vi "Quiz Scoreboard.vi"() -> ()   [LabVIEW 2025]
uses:
  Team.ctl
  State.ctl
  State Data.ctl
  <vilib>/DAQmx/create/channels.llb/DAQmx Create Channel (DI-Digital Input).vi
panel:
  out "Tab Control":enum32{"Setup", "Go"}(tab)
  in  "OK Button":bool
  in  "Team 1 Input":tag="Dev1/port0/line0" caption="Input"
  in  "Team 2 Input":tag="Dev1/port0/line1" caption="Input"
  in  "Team 3 Input":tag="Dev1/port0/line2" caption="Input"
  in  "Team 4 Input":tag="Dev1/port0/line3" caption="Input"
  in  "Team 1 Name":string="When I think about Yule I touch my Elf" caption="Team Name"
  in  "Team 2 Name":string="Bad Santa" caption="Team Name"
  in  "Team 3 Name":string="LabVIEWlots" caption="Team Name"
  in  "Team 4 Name":string="Operation Yule Tree" caption="Team Name"
  out "2D Picture":picture
  out "Team 4":T1
  out "Team 3":T1
  out "Team 2":T1
  out "Team 1":T1
  # "Team 1"
  # "Team 2"
  # "Team 3"
  # "Team 4"
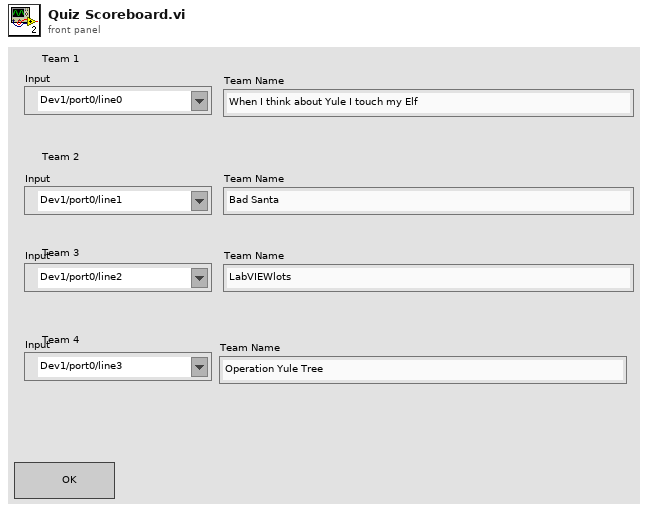
[diagram p1: front panel]
types:
  T1 = typedef "Team.ctl" = cluster{"ON":bool, "Name":bool, "Score":i32, "Split":string}
  T2 = typedef "State.ctl" = enum16{"Stop", "Initialize", "Wait for User Input", "Create DAQ Device"}
  T3 = typedef "State Data.ctl" = cluster{"Team 1":T1, "Team 2":T1, "Team 3":T1, "Team 4":T1, "Team Ref 1":refnum<vi>, "Team Ref 2":refnum<vi>, "Team Ref 3":refnum<vi>, "Team Ref 4":refnum<vi>, "Time":i32}
  T4 = typedef "eventvkey.ctl" = enum16{"ASCII", "Enter", "Return", "Shift", "Ctrl", "Alt", "Cmd", "Opt", "Caps", "NumLock", "Clear", "Break", "Up", "Down", "Left", "Right", "Insert", "Delete", "Home", "End", "PageUp", "PageDown", "Escape", "Help", "Pause", "ScrollLock", "F1", "F2", "F3", "F4", "F5", "F6", "F7", "F8", "F9", "F10", "F11", "F12", "F13", "F14", "F15", "F16", "F17", "F18", "F19", "F20", "F21", "F22", "F23", "F24", "Play", "VolumeUp", "VolumeDown", "Mute", "Two Byte Char"}
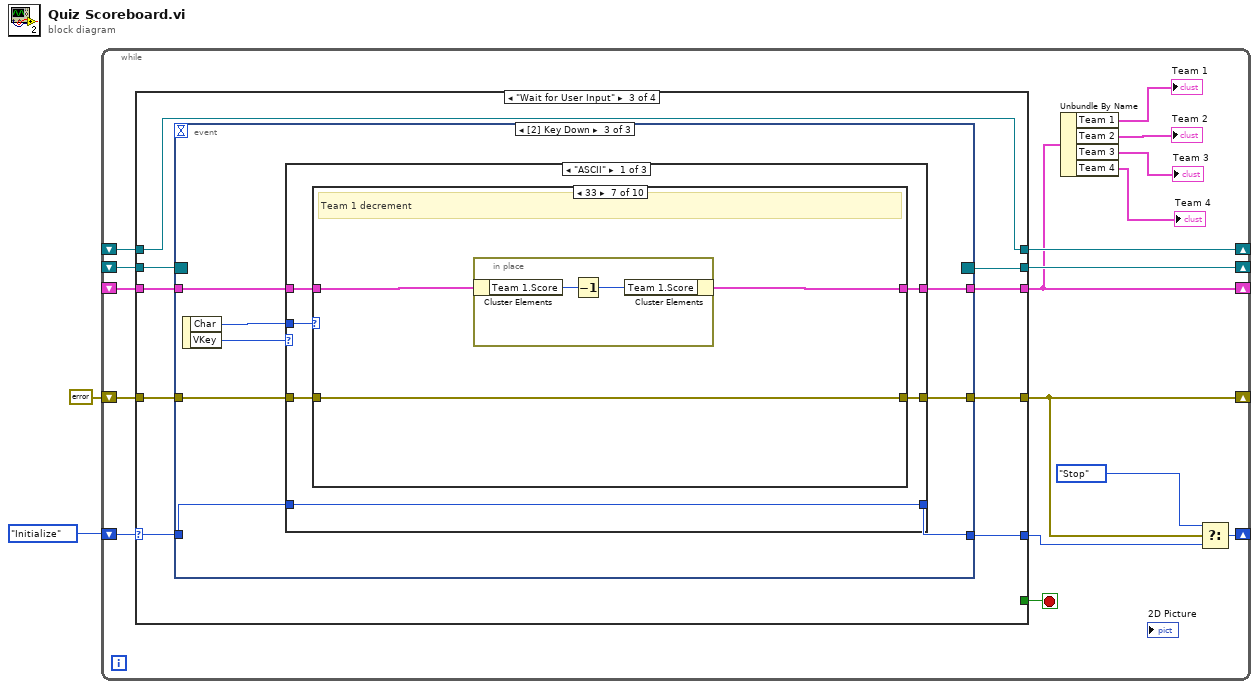
[diagram p0: block diagram]
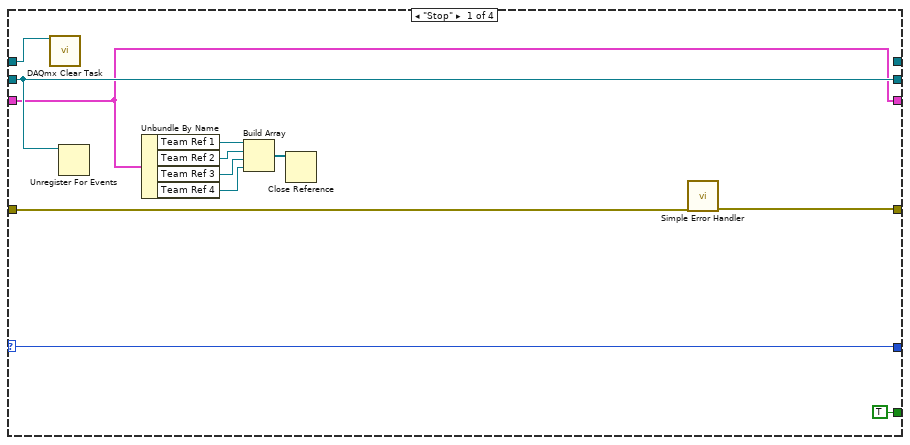
[diagram p2: hidden frame]
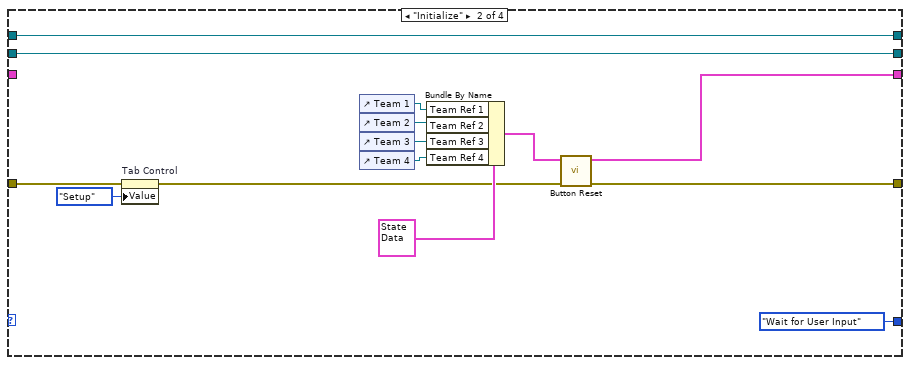
[diagram p3: hidden frame]
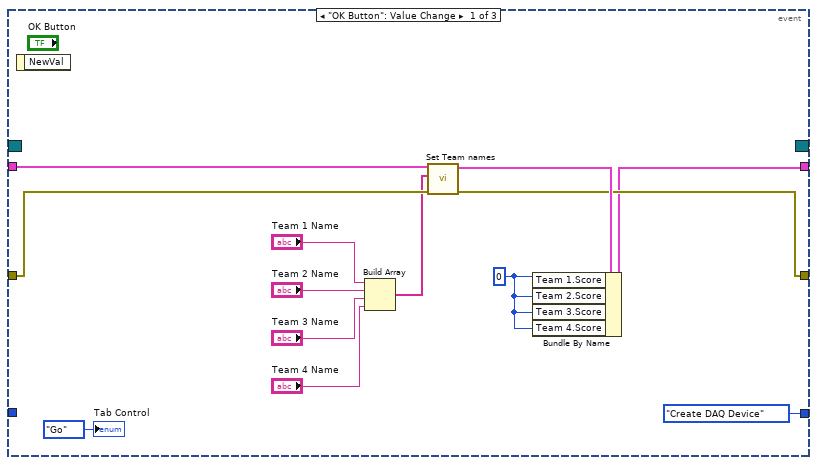
[diagram p4: hidden frame]
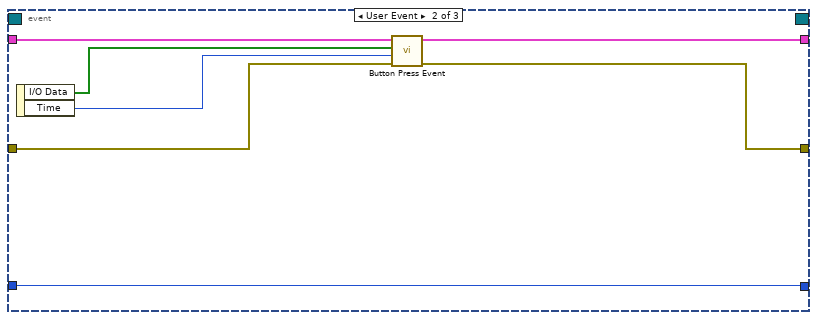
[diagram p5: hidden frame]
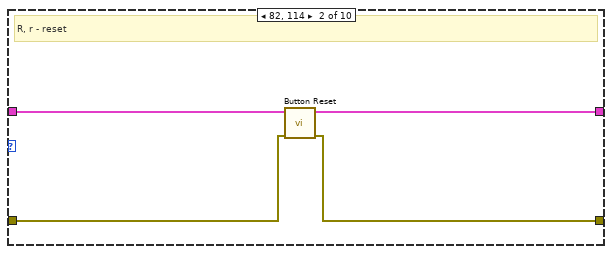
[diagram p7: hidden frame]
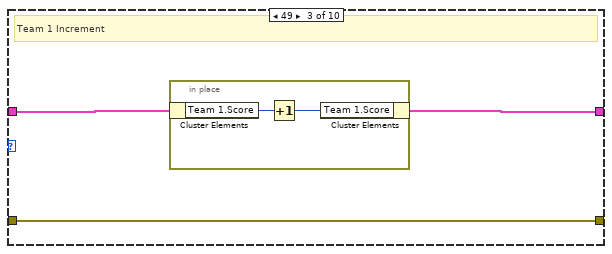
[diagram p8: hidden frame]
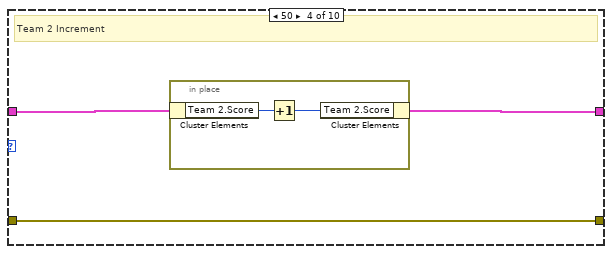
[diagram p9: hidden frame]
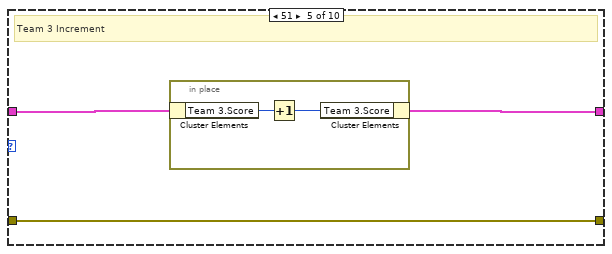
[diagram p10: hidden frame]
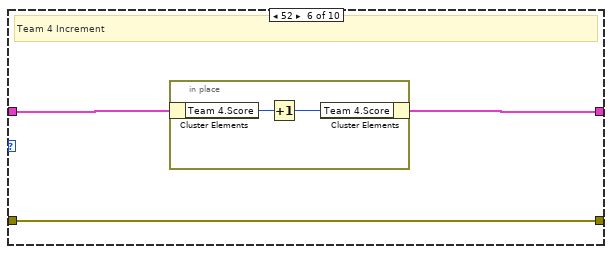
[diagram p11: hidden frame]
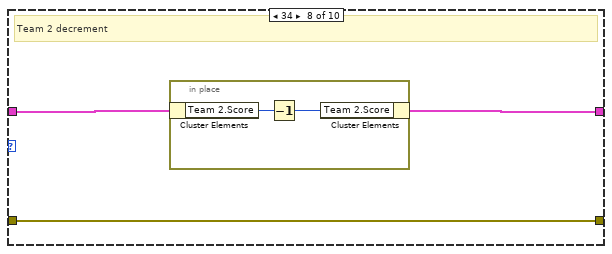
[diagram p12: hidden frame]
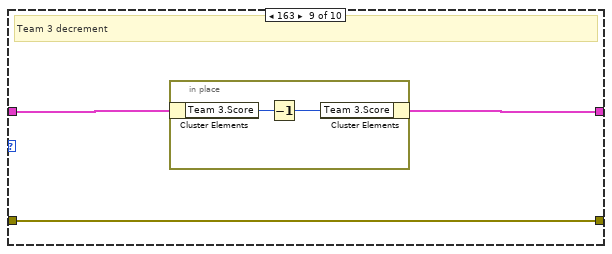
[diagram p13: hidden frame]
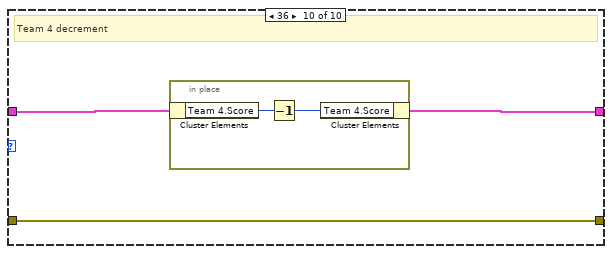
[diagram p14: hidden frame]
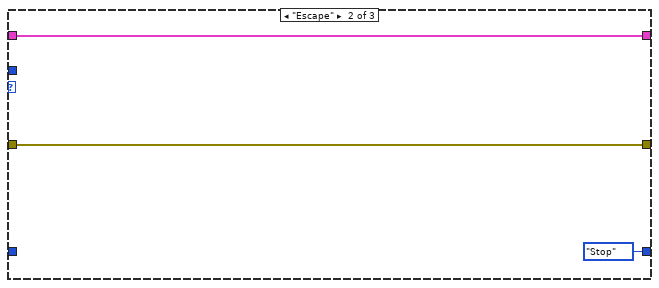
[diagram p15: hidden frame]
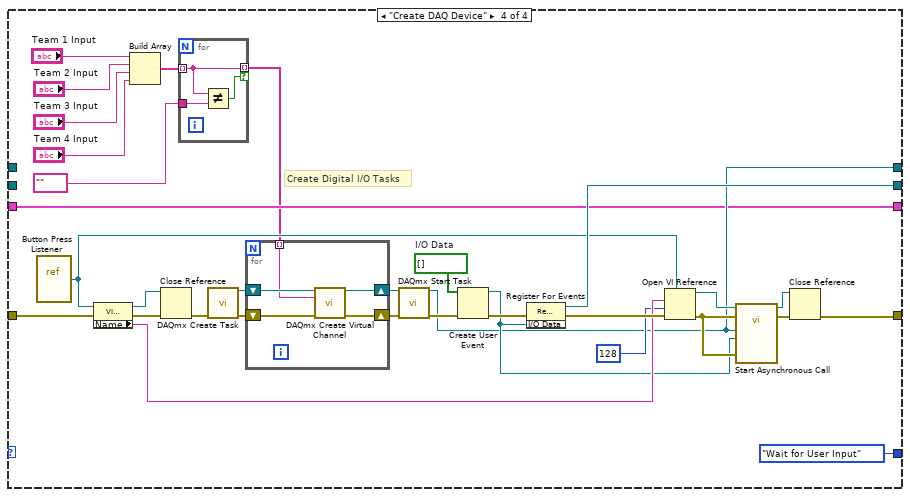
[diagram p17: hidden frame]
diagram:
  n1 = while {
    shift-right: [w14] -> _
    shift-left: State."Initialize" ("State") -> [w19]
    shift-right: [w16] -> _
    shift-left: errorcluster {"status"=FALSE, "code"=0, "source"=""} ("error out") -> [w18]
    shift-right: [w12] -> _
    shift-left: _ -> [w11]
    shift-right: [w10] -> _
    shift-left: _ -> [w9]
    shift-right: [w7] -> _
    shift-left: _ -> [w8]
    stop <- w17 stop-if-true
    n2 = case shown="\"Wait for User Input\"" w19 {
      selector: w19 -> [w30 _ w54 _]
      tunnel: [w30 State."Wait for User Input" ("State") w53 State."Wait for User Input" ("State")] -> w15
      tunnel: [w31 w32 w50 w149] -> w16
      tunnel: w18 -> [w20 w44 w51 w162]
      tunnel: [w28 w42 w52 w163] -> w12
      tunnel: [TRUE _ _ _] -> w17
      tunnel: w11 -> [w28 w42 w49 _]
      tunnel: [_ w41 w48 w145] -> w10
      tunnel: w9 -> [w27 w41 w48 _]
      tunnel: [w21 w33 w46 w144] -> w7
      tunnel: w8 -> [w21 _ w47 w144]
      frame "Stop" {
        n3 = call <vilib>:"DAQmx Clear Task.vi"("task in"=w27) -> ()  [unwired: 14 in, 1 out]
        n4 = Unregister For Events(event registration refnum=w28) -> ()  [unwired: 1 in, 1 out]
        n5 = Unbundle By Name(w21) -> ("Team Ref 1"=w26:refnum<vi>, "Team Ref 2"=w25:refnum<vi>, "Team Ref 3"=w24:refnum<vi>, "Team Ref 4"=w23:refnum<vi>)
        n6 = Build Array(w26, w25, w24, w23) -> (w22:refnum<vi>[])
        n7 = Close Reference(reference=w22) -> ()  [unwired: 1 in, 1 out]
        n8 = call <vilib>:"Simple Error Handler.vi"("error in (no error)"=w20) -> ("error out"=w31:errorcluster)  [unwired: 4 in, 4 out]
      }
      frame "Initialize" {
        n9 = property on="Tab Control" class="TabCtl (strict)"(error in=w44, "Value"=enum32{"Setup", "Go"}."Setup" ("Tab Control")) -> (error out=w34:errorcluster)  [unwired: 1 in, 1 out]
        n10 = control-ref of="Team 1"() -> (w39:refnum<vi>)
        n11 = control-ref of="Team 2"() -> (w38:refnum<vi>)
        n12 = control-ref of="Team 3"() -> (w37:refnum<vi>)
        n13 = control-ref of="Team 4"() -> (w36:refnum<vi>)
        n14 = Bundle By Name(cluster=T3 {"Team 1"={"ON"=FALSE, "Name"=FALSE, "Score"=0, "Split"=""}, "Team 2"={"ON"=FALSE, "Name"=FALSE, "Score"=0, "Split"=""}, "Team 3"={"ON"=FALSE, "Name"=FALSE, "Score"=0, "Split"=""}, "Team 4"={"ON"=FALSE, "Name"=FALSE, "Score"=0, "Split"=""}, "Team Ref 1"=refnum, "Team Ref 2"=refnum, "Team Ref 3"=refnum, "Team Ref 4"=refnum, "Time"=0} ("State Data"), "Team Ref 1"=w39, "Team Ref 2"=w38, "Team Ref 3"=w37, "Team Ref 4"=w36) -> (w35:T3)
        n15 = call "Button Reset.vi"("error in (no error)"=w34, "State Data in"=w35) -> ("error out"=w32:errorcluster, "State Data out"=w33:T3)  [unwired: 8 in]
      }
      frame "Wait for User Input" {
        n16 = event shown="[2] Key Down" {
          selector: w49 -> [_ _ _]
          dyn-events: [_ _ _] -> w52
          timeout: _ -> [_ _ _]
          tunnel: w54 -> [_ w74 w81]
          tunnel: [State."Create DAQ Device" ("State") w74 w80] -> w53
          tunnel: w51 -> [w64 w72 w79]
          tunnel: [w62 w71 w78] -> w50
          tunnel: w47 -> [w65 w70 w76]
          tunnel: [w56 w69 w75] -> w46
          event "OK Button": Value Change {
            w55 = 0 ("Team 1.Score")
            n17 = event-data() -> ()  [unwired: 1 in, 1 out]
            n18 = Build Array("Team 1 Name", "Team 2 Name", "Team 3 Name", "Team 4 Name") -> (w58:string[])
            n19 = call "Set Team names.vi"("error in (no error)"=w64, "Names"=w58, "State Data in"=w65) -> ("error out"=w62:errorcluster, "State Data out"=w63:T3)  [unwired: 7 in]
            n20 = Bundle By Name(cluster=w63, "Team 1.Score"=w55, "Team 2.Score"=w55, "Team 3.Score"=w55, "Team 4.Score"=w55) -> (w56:T3)
            "Tab Control" <- enum32{"Setup", "Go"}."Go" ("Tab Control")
          }
          event User Event {
            n21 = event-data() -> ("I/O Data"=w73:bool[], "Time"=w68:u32)  [unwired: 1 in]
            n22 = call "Button Press Event.vi"("error in (no error)"=w72, "Event Time"=w68, "Buttons"=w73, "State Data in"=w70) -> ("error out"=w71:errorcluster, "State Data out"=w69:T3)  [unwired: 6 in]
          }
          event Key Down {
            n23 = event-data() -> ("Char"=w77:i16, "VKey"=w82:T4)  [unwired: 1 in]
            n24 = case shown="\"ASCII\"" w82 {
              tunnel: w81 -> [w88 _ w140]
              tunnel: [w88 State."Stop" ("State") w140] -> w80
              tunnel: w79 -> [w85 w137 w139]
              tunnel: [w83 w137 w139] -> w78
              tunnel: w77 -> [w87 _ _]
              tunnel: w76 -> [w86 w135 w138]
              tunnel: [w84 w135 w138] -> w75
              frame "ASCII" {
                n25 = case shown="33" w87 {
                  tunnel: w86 -> [w90 w94 w97 w102 w107 w112 w117 w122 w127 w132]
                  tunnel: w85 -> [w89 w93 w95 w100 w105 w110 w115 w120 w125 w130]
                  tunnel: [w90 w92 w96 w101 w106 w111 w116 w121 w126 w131] -> w84
                  tunnel: [w89 w91 w95 w100 w105 w110 w115 w120 w125 w130] -> w83
                  frame Default {
                  }
                  frame 82, 114 {
                    # "R, r - reset"
                    n26 = call "Button Reset.vi"("error in (no error)"=w93, "State Data in"=w94) -> ("error out"=w91:errorcluster, "State Data out"=w92:T3)  [unwired: 8 in]
                  }
                  frame 49 {
                    # "Team 1 Increment"
                    n27 = in-place {
                      n28 = in-place-cluster #1(w97) -> ("Team 1.Score"=w99:i32)
                      n29 = Increment(x=w99) -> (x+1=w98:i32)
                      n30 = in-place-cluster #1("Team 1.Score"=w98) -> (w96:T3)
                    }
                  }
                  frame 50 {
                    # "Team 2 Increment"
                    n31 = in-place {
                      n32 = in-place-cluster #2(w102) -> ("Team 2.Score"=w104:i32)
                      n33 = Increment(x=w104) -> (x+1=w103:i32)
                      n34 = in-place-cluster #2("Team 2.Score"=w103) -> (w101:T3)
                    }
                  }
                  frame 51 {
                    # "Team 3 Increment"
                    n35 = in-place {
                      n36 = in-place-cluster #3(w107) -> ("Team 3.Score"=w109:i32)
                      n37 = Increment(x=w109) -> (x+1=w108:i32)
                      n38 = in-place-cluster #3("Team 3.Score"=w108) -> (w106:T3)
                    }
                  }
                  frame 52 {
                    # "Team 4 Increment"
                    n39 = in-place {
                      n40 = in-place-cluster #4(w112) -> ("Team 4.Score"=w114:i32)
                      n41 = Increment(x=w114) -> (x+1=w113:i32)
                      n42 = in-place-cluster #4("Team 4.Score"=w113) -> (w111:T3)
                    }
                  }
                  frame 33 {
                    # "Team 1 decrement"
                    n43 = in-place {
                      n44 = in-place-cluster #5(w117) -> ("Team 1.Score"=w119:i32)
                      n45 = Decrement(x=w119) -> (x-1=w118:i32)
                      n46 = in-place-cluster #5("Team 1.Score"=w118) -> (w116:T3)
                    }
                  }
                  frame 34 {
                    # "Team 2 decrement"
                    n47 = in-place {
                      n48 = in-place-cluster #6(w122) -> ("Team 2.Score"=w124:i32)
                      n49 = Decrement(x=w124) -> (x-1=w123:i32)
                      n50 = in-place-cluster #6("Team 2.Score"=w123) -> (w121:T3)
                    }
                  }
                  frame 163 {
                    # "Team 3 decrement"
                    n51 = in-place {
                      n52 = in-place-cluster #7(w127) -> ("Team 3.Score"=w129:i32)
                      n53 = Decrement(x=w129) -> (x-1=w128:i32)
                      n54 = in-place-cluster #7("Team 3.Score"=w128) -> (w126:T3)
                    }
                  }
                  frame 36 {
                    # "Team 4 decrement"
                    n55 = in-place {
                      n56 = in-place-cluster #8(w132) -> ("Team 4.Score"=w134:i32)
                      n57 = Decrement(x=w134) -> (x-1=w133:i32)
                      n58 = in-place-cluster #8("Team 4.Score"=w133) -> (w131:T3)
                    }
                  }
                }
              }
              frame "Escape" {
              }
              frame Default {
              }
            }
          }
        }
      }
      frame "Create DAQ Device" {
        w165 = bool[] []  # I/O Data
        # "Create Digital I/O Tasks"
        n59 = vi-ref "Button Press Listener.vi"() -> (w156:refnum<vi>)
        n60 = property class="VI (strict)"(reference=w156, error in=w162) -> (reference out=w161:refnum<vi>, error out=w160:errorcluster, "Name"=w157:string)
        n61 = Build Array("Team 1 Input", "Team 2 Input", "Team 3 Input", "Team 4 Input") -> (w143:tag[])
        n62 = Close Reference(reference=w161, error in (no error)=w160) -> (error out=w159:errorcluster)
        n63 = for {
          tunnel: w143 -> [w174] mode=indexing
          tunnel: tag "" ("Team 1 Input 2") -> [w175]
          tunnel: [w174] -> w141 mode=indexing if=w173
          n64 = Not Equal?(x=w174, y=w175) -> (x != y?=w173:bool)
        }
        n65 = call <vilib>:"DAQmx Create Task.vi"("error in"=w159) -> ("task out"=w171:refnum<k21>, "error out"=w172:errorcluster)  [unwired: 13 in]
        n66 = for {
          shift-right: [w178] -> w153
          shift-left: w171 -> [w179]
          shift-right: [w177] -> w148
          shift-left: w172 -> [w180]
          tunnel: w141 -> [w176] mode=indexing
          n67 = call-poly <vilib>:"DAQmx Create Virtual Channel.vi"("task in"=w179, "lines"=w176, "error in"=w180) -> ("task out"=w178:refnum<k21>, "error out"=w177:errorcluster)  [unwired: 11 in]
        }
        n68 = call <vilib>:"DAQmx Start Task.vi"("task/channels in"=w153, "error in"=w148) -> ("task out"=w145:refnum<k21>, "error out"=w147:errorcluster)  [unwired: 12 in]
        n69 = Create User Event(user event datatype=w165, error in=w147) -> (user event=w152:refnum<user-event>, error out=w164:errorcluster)
        n70 = register-events(error in=w164, w152) -> (reference out=w163:refnum<event-registration>, error out=w158:errorcluster)  [unwired: 1 in]
        n71 = Open VI Reference(type specifier VI Refnum (for type only)=w156, vi path=w157, options=128, error in (no error)=w158) -> (vi reference=w155:refnum<vi>, error out=w154:errorcluster)  [unwired: 2 in]
        n72 = call-by-ref "Start Asynchronous Call"(reference=w155, error in=w154, 8:"error in (no error)"=w154, "I/O Data"=w152, "DaqMX task"=w145) -> (reference out=w151:refnum<vi>, error out=w150:errorcluster)  [unwired: 9 in]
        n73 = Close Reference(reference=w151, error in (no error)=w150) -> (error out=w149:errorcluster)
      }
    }
    n74 = Unbundle By Name(w7) -> ("Team 1"=→"Team 1":T1, "Team 2"=→"Team 2":T1, "Team 3"=→"Team 3":T1, "Team 4"=→"Team 4":T1)
    n75 = Select(t=State."Stop" ("State"), s=w16, f=w15) -> (s? t:f=w14:T2)
  }
